vi "NI VeriStand - Rename Custom Device Item.vi"(7 "Force Rename (F)":bool, 8 "error in (no error)":errorcluster, 10 "New Name":string, 11 "Item Ref in":T1 format="%.0x") -> (0 "error out":errorcluster, 2 "Request invalid?":bool, 3 "Item Ref out":T1 format="%.0x")   [LabVIEW 2020, in "Custom Device API.lvlib"]
doc: "Applies a <B>New Name</B> to the item specified by <B>Item Ref in</B>. If the <B>New Name</B> you specify already exists in the same section, this VI does nothing and the <B>Request invalid?</B> indicator returns TRUE."
uses:
  <vilib>/NI VeriStand/Custom Device API/Custom Device API.lvlib
  <vilib>/NI VeriStand/Custom Device API/Custom Device Item Ref.ctl
  a0b4c00c-b8d7-46a5-9e6e-b1a652cbf596.vi
  <vilib>/NI VeriStand/Custom Device API/Custom Device Offline Path.vi
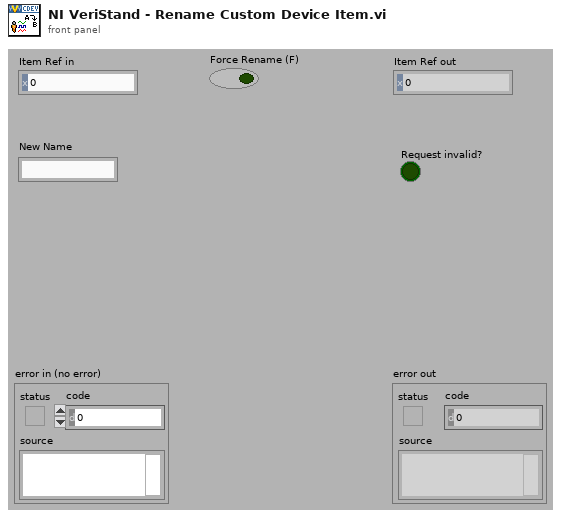
[diagram p1: front panel]
types:
  T1 = typedef "Custom Device API.lvlib/Custom Device Item Ref.ctl" = u64
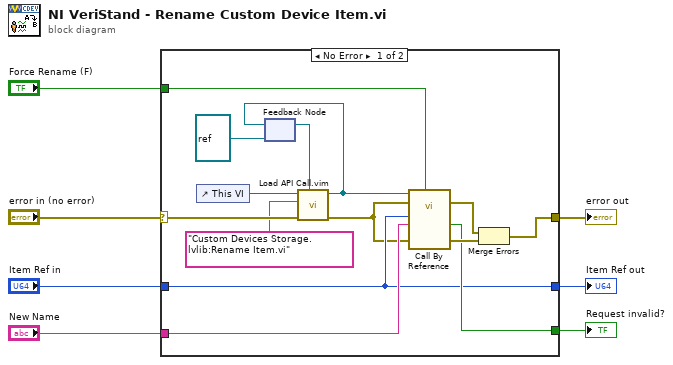
[diagram p0: block diagram]
diagram:
  n1 = case shown="No Error" "error in (no error)" {
    selector: "error in (no error)" -> [w13 w23]
    tunnel: [w20 w23] -> w7
    tunnel: "Item Ref in" -> [w16 w22]
    tunnel: "New Name" -> [w19 _]
    tunnel: [w16 w22] -> w4
    tunnel: [w18 _] -> w3
    tunnel: "Force Rename (F)" -> [w17 _]
    frame No Error {
      n2 = control-ref of="This VI"() -> (w14:refnum<vi>)
      n3 = feedback #1(refnum<vi> refnum ("type specifier VI Refnum (for type only)")) -> (w15:refnum<vi>)
      n4 = call "Load API Call.vim"("VI reference in"=w15, "error in (no error)"=w13, "VI qualified name"="Custom Devices Storage.lvlib:Rename Item.vi", "Caller VI ref"=w14) -> ("error out"=w11:errorcluster, "VI reference"=w12:refnum<vi>)  [unwired: 6 in]
      n5 = feedback-in #1(w12) -> ()
      n6 = call-by-ref "?"(reference=w12, error in=w11, "Force Rename? (F)"=w17, 8:"error in (no error)"=w11, "New Name"=w19, "Item Ref in"=w16) -> (error out=w8:errorcluster, 0:"error out"=w21:errorcluster, "Request invalid?"=w18:bool)  [unwired: 5 in, 2 out]
      n7 = Merge Errors(w8, w21) -> (w20:errorcluster)
    }
    frame Error {
    }
  }
  "Item Ref out" <- w4
  "error out" <- w7
  "Request invalid?" <- w3
